vi "Create Serial Output Channel I2C IO x4.vi"() -> (4 "serial output channel i2c io x4":T2)   [LabVIEW 2023, in "GettingStarted_Common_148X_FPGA.lvlib"]
uses:
  GettingStarted_Common_148X_FPGA.lvlib
  Types/I2C IO.ctl
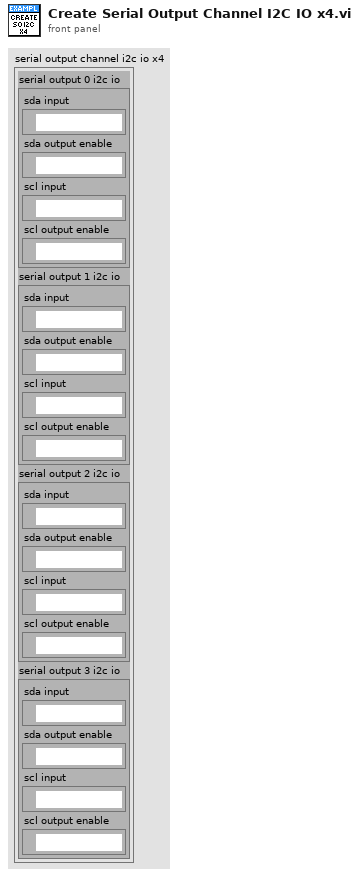
[diagram p1: front panel]
types:
  T1 = typedef "GettingStarted_Common_148X_FPGA.lvlib/I2C IO.ctl" = cluster{"sda input":refnum<k21>, "sda output enable":refnum<k21>, "scl input":refnum<k21>, "scl output enable":refnum<k21>}
  T2 = cluster{"serial output 0 i2c io":T1, "serial output 1 i2c io":T1, "serial output 2 i2c io":T1, "serial output 3 i2c io":T1}
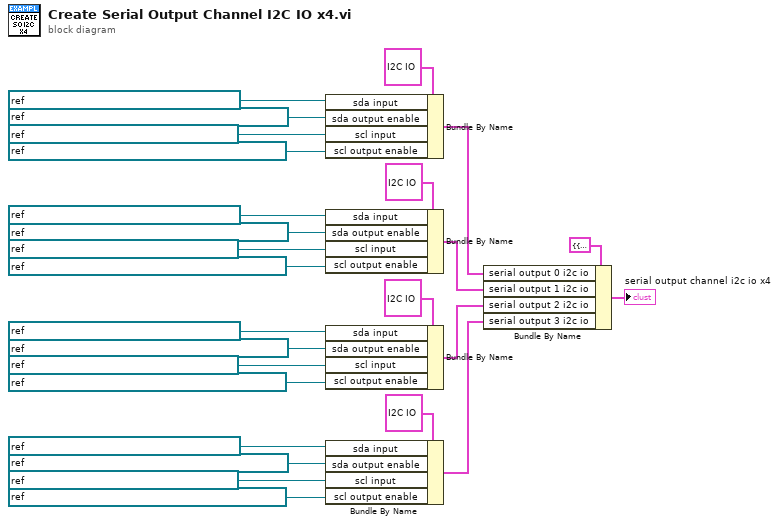
[diagram p0: block diagram]
diagram:
  n1 = Bundle By Name(cluster=T1 {"sda input"="IO Socket\\SI 0 Deserializer I2C SDA Input", "sda output enable"="IO Socket\\SI 0 Deserializer I2C SDA Output Enable", "scl input"="IO Socket\\SI 0 Deserializer I2C SCL Input", "scl output enable"="IO Socket\\SI 0 Deserializer I2C SCL Output Enable"}, "sda input"=refnum<k21> "IO Socket\\SO 0 Serializer I2C SDA Input", "sda output enable"=refnum<k21> "IO Socket\\SO 0 Serializer I2C SDA Output Enable", "scl input"=refnum<k21> "IO Socket\\SO 0 Serializer I2C SCL Input", "scl output enable"=refnum<k21> "IO Socket\\SO 0 Serializer I2C SCL Output Enable") -> (w5:T1)
  n2 = Bundle By Name(cluster=T1 {"sda input"="IO Socket\\SI 0 Deserializer I2C SDA Input", "sda output enable"="IO Socket\\SI 0 Deserializer I2C SDA Output Enable", "scl input"="IO Socket\\SI 0 Deserializer I2C SCL Input", "scl output enable"="IO Socket\\SI 0 Deserializer I2C SCL Output Enable"}, "sda input"=refnum<k21> "IO Socket\\SO 1 Serializer I2C SDA Input", "sda output enable"=refnum<k21> "IO Socket\\SO 1 Serializer I2C SDA Output Enable", "scl input"=refnum<k21> "IO Socket\\SO 1 Serializer I2C SCL Input", "scl output enable"=refnum<k21> "IO Socket\\SO 1 Serializer I2C SCL Output Enable") -> (w2:T1)
  n3 = Bundle By Name(cluster=T1 {"sda input"="IO Socket\\SI 0 Deserializer I2C SDA Input", "sda output enable"="IO Socket\\SI 0 Deserializer I2C SDA Output Enable", "scl input"="IO Socket\\SI 0 Deserializer I2C SCL Input", "scl output enable"="IO Socket\\SI 0 Deserializer I2C SCL Output Enable"}, "sda input"=refnum<k21> "IO Socket\\SO 2 Serializer I2C SDA Input", "sda output enable"=refnum<k21> "IO Socket\\SO 2 Serializer I2C SDA Output Enable", "scl input"=refnum<k21> "IO Socket\\SO 2 Serializer I2C SCL Input", "scl output enable"=refnum<k21> "IO Socket\\SO 2 Serializer I2C SCL Output Enable") -> (w3:T1)
  n4 = Bundle By Name(cluster=T1 {"sda input"="IO Socket\\SI 0 Deserializer I2C SDA Input", "sda output enable"="IO Socket\\SI 0 Deserializer I2C SDA Output Enable", "scl input"="IO Socket\\SI 0 Deserializer I2C SCL Input", "scl output enable"="IO Socket\\SI 0 Deserializer I2C SCL Output Enable"}, "sda input"=refnum<k21> "IO Socket\\SO 3 Serializer I2C SDA Input", "sda output enable"=refnum<k21> "IO Socket\\SO 3 Serializer I2C SDA Output Enable", "scl input"=refnum<k21> "IO Socket\\SO 3 Serializer I2C SCL Input", "scl output enable"=refnum<k21> "IO Socket\\SO 3 Serializer I2C SCL Output Enable") -> (w4:T1)
  n5 = Bundle By Name(cluster=T2 {"serial output 0 i2c io"={"sda input"="IO Socket\\SI 0 Deserializer I2C SDA Input", "sda output enable"="IO Socket\\SI 0 Deserializer I2C SDA Output Enable", "scl input"="IO Socket\\SI 0 Deserializer I2C SCL Input", "scl output enable"="IO Socket\\SI 0 Deserializer I2C SCL Output Enable"}, "serial output 1 i2c io"={"sda input"="IO Socket\\SI 0 Deserializer I2C SDA Input", "sda output enable"="IO Socket\\SI 0 Deserializer I2C SDA Output Enable", "scl input"="IO Socket\\SI 0 Deserializer I2C SCL Input", "scl output enable"="IO Socket\\SI 0 Deserializer I2C SCL Output Enable"}, "serial output 2 i2c io"={"sda input"="IO Socket\\SI 0 Deserializer I2C SDA Input", "sda output enable"="IO Socket\\SI 0 Deserializer I2C SDA Output Enable", "scl input"="IO Socket\\SI 0 Deserializer I2C SCL Input", "scl output enable"="IO Socket\\SI 0 Deserializer I2C SCL Output Enable"}, "serial output 3 i2c io"={"sda input"="IO Socket\\SI 0 Deserializer I2C SDA Input", "sda output enable"="IO Socket\\SI 0 Deserializer I2C SDA Output Enable", "scl input"="IO Socket\\SI 0 Deserializer I2C SCL Input", "scl output enable"="IO Socket\\SI 0 Deserializer I2C SCL Output Enable"}} ("serial output channel i2c io x4"), "serial output 0 i2c io"=w5, "serial output 1 i2c io"=w2, "serial output 2 i2c io"=w3, "serial output 3 i2c io"=w4) -> (→"serial output channel i2c io x4":T2)
